vi "GetType.vi"(8 "error in (no error)":errorcluster, 11 "Configure Relays Msg":refnum<class "Configure Relays Msg.lvclass">) -> (0 "error out":errorcluster, 2 "Data Sample":variant, 3 "Configure Relays Msg":refnum<class "Configure Relays Msg.lvclass">)   [LabVIEW 2015, in "LS218.lvlib" / "Configure Relays Msg.lvclass"]
uses:
  Configure Relays Msg.lvclass
  Configure Relays Msg.lvclass/Configure Relays Msg.ctl
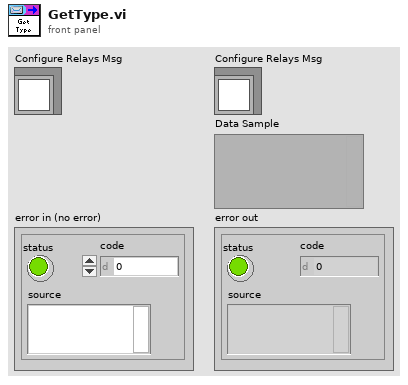
[diagram p1: front panel]
types:
  T1 = cluster{"Relay (0)":i32, "Input (0)":i32, "Mode (0:Off)":enum16{"Off", "On", "Alarms"}, "Alarm Type (0:Low)":u16}
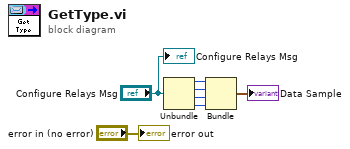
[diagram p0: block diagram]
diagram:
  n1 = Unbundle("Configure Relays Msg") -> (w4:i32, w3:i32, w2:enum16{"Off", "On", "Alarms"}, w1:u16)
  n2 = Bundle("Relay (0)"=w4, "Input (0)"=w3, "Mode (0:Off)"=w2, "Alarm Type (0:Low)"=w1) -> (→"Data Sample":T1)  [unwired: 1 in]
  "error out" <- "error in (no error)"
  "Configure Relays Msg" <- "Configure Relays Msg"
